vi "CMI Sync V3 Error Check.vi"(8 "error in":errorcluster, 11 "VISA in":refnum<visa-resource-name>) -> (0 "error out":errorcluster, 2 "error string":string, 3 "VISA out":refnum<visa-resource-name>)   [LabVIEW 2020, in "AWG.lvlib" / "CMI Sync Unit V3.lvlib"]
doc: "Check if there is an error in the sync unit error buffer."
uses:
  CMI Sync Unit V3.lvlib
  <vilib>/Utility/error.llb/Error Cluster From Error Code.vi
  <vilib>/ErrorRing/Error Ring.xnode
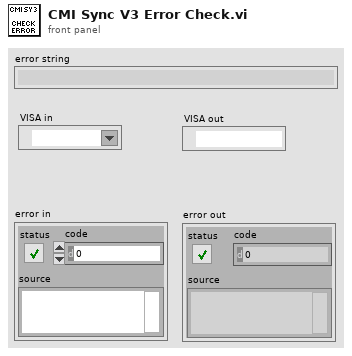
[diagram p1: front panel]
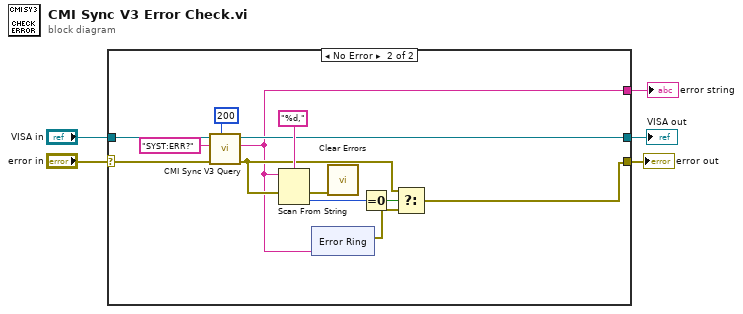
[diagram p0: block diagram]
diagram:
  n1 = case shown="No Error" "error in" {
    selector: "error in" -> [w7 w20]
    tunnel: "VISA in" -> [w6 w19]
    tunnel: [w6 w10] -> w4
    tunnel: [w7 w11] -> w2
    tunnel: [_ w9] -> w1
    frame Error {
    }
    frame No Error {
      n2 = call "CMI Sync V3 Query.vi"("read byte count (100)"=u32 200, "error in"=w20, "command"="SYST:ERR?", "VISA in"=w19) -> ("error out"=w13:errorcluster, "read buffer"=w9:string, "VISA resource name out"=w10:refnum<visa-resource-name>)  [unwired: 5 in]
      n3 = Scan From String(format string="%d,", input string=w9, error in=w13) -> (error out=w8:errorcluster, output 1=w15:i32)  [unwired: 2 in, 2 out]
      n4 = xnode "Error Ring"("parameter 0"=w9) -> ("error out"=w12:errorcluster)
      n5 = call <vilib>:"Clear Errors.vi"("error in (no error)"=w8) -> ()  [unwired: 5 in, 2 out]
      n6 = Equal To 0?(x=w15) -> (x = 0?=w14:bool)
      n7 = Select(t=w13, s=w14, f=w12) -> (s? t:f=w11:errorcluster)
    }
  }
  "error out" <- w2
  "VISA out" <- w4
  "error string" <- w1
